vi "Read Station status.vi"(8 "error in (no error)":errorcluster, 11 "Fiber Auto Collimation state data in":refnum<class "Fiber Auto Collimation state data.lvclass">) -> (0 "error out":errorcluster, 2 "Station status":T1, 3 "Fiber Auto Collimation state data out":refnum<class "Fiber Auto Collimation state data.lvclass">)   [LabVIEW 2018, in "Fiber Auto Collimation state data.lvclass"]
doc: "The main purpose of these states is to define the appearance (or lack thereof) of the main VI's front panel.\n\nThe default template is set up so that when \"Running\" the main window will be hidden, with asynchronous panels having been launched to handle all UI and other needs.\n\nIn the other states, the default template will be visible with a short message indicating the current status.\n\nThe above may change based on the needs of stations derived from the template, and other options may be added as well."
uses:
  Fiber Auto Collimation state data.lvclass
  Station status.ctl
  Fiber Auto Collimation state data.lvclass/Fiber Auto Collimation state data.ctl
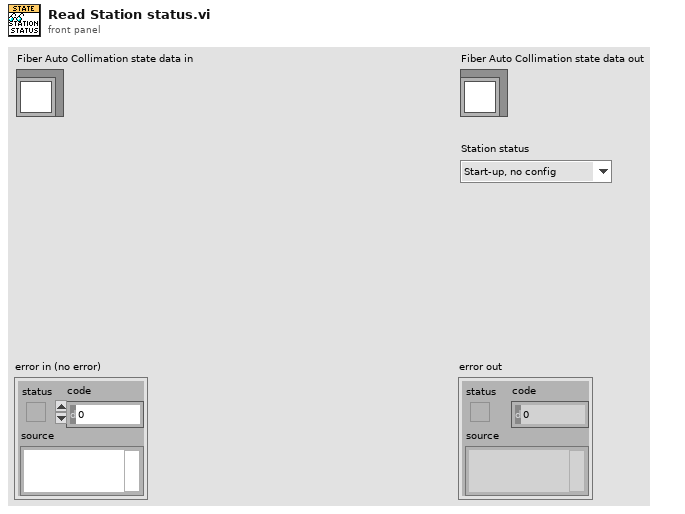
[diagram p1: front panel]
types:
  T1 = typedef "Fiber Auto Collimation state data.lvclass/Station status.ctl" = enum16{"Start-up, no config", "Start-up, config loaded", "Start-up, config problem", "Running", "Shutting down"}
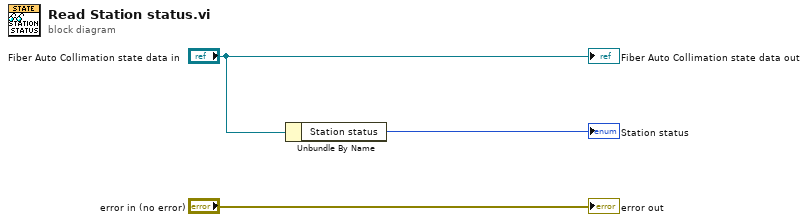
[diagram p0: block diagram]
diagram:
  n1 = Unbundle By Name("Fiber Auto Collimation state data in") -> ("Station status"=→"Station status":T1)
  "error out" <- "error in (no error)"
  "Fiber Auto Collimation state data out" <- "Fiber Auto Collimation state data in"
